vi "ResponseParase.vi"(8 "error in (no error)":errorcluster, 11 "input string":string) -> (0 "error out":errorcluster, 2 "error code":i32, 3 "OutputArray":string[](array[string]))   [LabVIEW 2015]
uses:
  <vilib>/regexp/Match Regular Expression.xnode
panel:
  out "element":string
  in  "regular expression":string=",+-?\\w*\\s*\\w*"
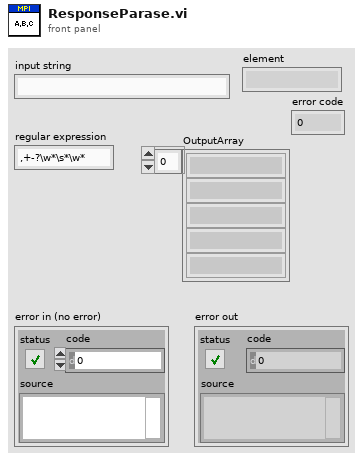
[diagram p1: front panel]
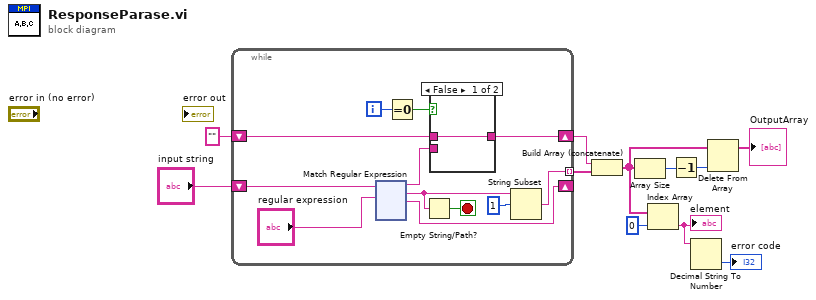
[diagram p0: block diagram]
diagram:
  n1 = while {
    shift-right: [w22] -> _
    shift-left: "input string" -> [w21]
    shift-right: [w16] -> w9
    shift-left: "" ("before match") -> [w15]
    tunnel: [w13] -> w8 mode=indexing
    i -> [w19]
    stop <- w23 stop-if-true
    n2 = xnode ("Match Regular Expression")("input string"=w21, "regular expression"="regular expression") -> ("before match"=w17:string, "whole match"=w14:string, "after match"=w22:string)  [unwired: 4 in, 2 out]
    n3 = Equal To 0?(x=w19) -> (x = 0?=w18:bool)
    n4 = Empty String/Path?(string/path=w14) -> (empty?=w23:bool)
    n5 = case shown="False" w18 {
      tunnel: [w24 w25] -> w16
      tunnel: w17 -> [_ w25]
      tunnel: w15 -> [w24 _]
      frame False {
      }
      frame True {
      }
    }
    n6 = String Subset(string=w14, offset (0)=1 ("length (rest)")) -> (substring=w13:string)  [unwired: 1 in]
  }
  n7 = Build Array (concatenate)(w9, w8) -> (w4:string[])
  n8 = Array Size(array=w4) -> (size(s)=w6:i32)
  n9 = Index Array(array=w4, index=0) -> (element=w2:string)
  "element" <- w2
  n10 = Decrement(x=w6) -> (x-1=w5:i32)
  n11 = Decimal String To Number(string=w2) -> (number=→"error code":i32)  [unwired: 2 in, 1 out]
  n12 = Delete From Array(array=w4, index=w5) -> (array with subset deleted=→"OutputArray":string[])  [unwired: 1 in, 1 out]
